vi "DefesaAntigaAdaptada.vi"(0 "Our Robot":T1={"id"=0, "function"=enum."Attacker", "x"=0.0, "y"=0.0, "orientation"=0.0, "v_tangent"=0.0, "v_normal"=0.0, "v_ang"=0.0, "kick_x"=0.0, "kick_z"=0.0, "dribble"=FALSE, "Timestamp"=timestamp(0 s since 1904-01-01), "estimatives"={"est_v_tangent"=0.0, "est_v_normal"=0.0, "est_vx"=0.0, "est_vy"=0.0, "Pos Robot Est"=[]}, "dest_x_kick"=0.0, "dest_y_kick"=0.0, "Gap Coord"=[], "States"=enum."GoToTangent", "Path "=[], "Path  Smooth"=[], "Dest"=[]}, 1 "total de \ndefensores":i32, 2 "Id duelist":u32, 3 "Stop?":bool=TRUE, 4 "AI Parameters":T12={"GotoKick"={"Dist do cone a frente"=150.0, "attacker farback"=1500.0, "Perto"=300.0, "min dist to kick"=150.0, "kick eps"=0.0, "Time to transition"=0.05}, "Attacker"={"CC chute"=0.09, "CC passe"=0.045, "Kick Force"=100.0, "ball-robot Kick"=200.0, "ball-robot Pass"=0.3, "drible\nAttk"=FALSE}, "Defender"={"D max"=1700.0, "Vel p/ robô av"=1000.0, "Kick Force"=100.0, "D atk-def"=0.0, "D farback"=0.0, "drible\ndef"=FALSE, "drible\ngoalie"=FALSE}, "Timeout"={"Field/v in x"=6.0, "Dist Robots"=300, "Dist up in y"=300}, "Pose Striker"={"dist"=200.0, "Numeric"=-4.0, "dist 2"=200.0, "drible\nstriker"=FALSE}, "Dist Stop"=300.0, "D ball out"=200, "D central gap "=150.0, "T pass"=0.0, "Force ++"=0.0, "range kick"=0.0, "Chute alto"=TRUE, "Marcador novo"=TRUE, "drible"=FALSE, "D drible"=300.0, "Versão Striker"=enum."Auto", "Defesa"=enum."ManMark", "Marcador"=enum."Marcar Segndo mais perigoso", "Receptor passe"=enum."Auto", "Área"=enum."Quadrada"} {"D drible" format="%#_13g"; "D central gap" format="%#_13g"; "Dist Stop" format="%#_13g"; "Pose Striker"."Numeric" format="%#_13g"; "Defender"."Kick Force" format="%#_13g"; "Defender"."Vel p/ robô av" format="%#_13g"; "Attacker"."ball-robot Kick" format="%#_13g"; "Attacker"."Kick Force" format="%#_13g"; "Attacker"."CC passe" format="%#_13g"; "Attacker"."CC chute" format="%#_13g"; "GotoKick"."kick eps" format="%#_13g"; "GotoKick"."min dist to kick" format="%#_13g"; "GotoKick"."Perto" format="%#_13g"; "GotoKick"."attacker farback" format="%#_13g"; "GotoKick"."Dist do cone a frente" format="%#_13g"}, 5 "balls":T7[](array[typedef]), 9 "geometry":T8, 10 "Atacando contra?":bool=TRUE, 11 "Field defense":dbl[](array[numeric]), 12 "Defensores":u32[](array[numeric]), 14 "IA State Input 2":T6={"our_robots"=[], "enemy_robots"=[], "balls"=[], "geometry"={"line_width"=0, "field_length"=0, "field_width"=0, "boundary_width"=0, "referee_width"=0, "goal_width"=0, "goal_depth"=0, "goal_wall_width"=0, "center_circle_radius"=0, "defense_radius"=0, "defense_stretch"=0, "free_kick_from_defense_dist"=0, "penalty_spot_from_field_line_dist"=0, "penalty_line_from_spot_dist"=0}, "IA Judge"={"stage"="", "command"="", "our_goalie_id"=0.0, "enemy_goalie_id"=0.0, "command enum"=enum."Halt", "Time"=enum."Azul"}, "Received Timestamp"=timestamp(0 s since 1904-01-01), "Events"={"Touch"=FALSE, "Ball out"=FALSE, "id touch"=0.0, "Ball out of \nVision"=FALSE, "Ball inside \nGoalie area"=FALSE, "Robot not responding"=FALSE, "Robots responding status"=[1.0, 1.0, 1.0, 1.0, 1.0, 1.0], "Enemy Ball \nPossession"=FALSE, "Pass State"=FALSE, "id end of pass"=0.0, "Kick"=FALSE, "Id ini Possession"=0.0, "Ball Possesion"=FALSE, "Id Possesion"=0.0, "Direct Kick"=FALSE, "2nd Strk Ativo"=FALSE}}) -> (6 "Robot out":T1={"id"=0, "function"=enum."Attacker", "x"=0.0, "y"=0.0, "orientation"=0.0, "v_tangent"=0.0, "v_normal"=0.0, "v_ang"=0.0, "kick_x"=0.0, "kick_z"=0.0, "dribble"=FALSE, "Timestamp"=timestamp(0 s since 1904-01-01), "estimatives"={"est_v_tangent"=0.0, "est_v_normal"=0.0, "est_vx"=0.0, "est_vy"=0.0, "Pos Robot Est"=[]}, "dest_x_kick"=0.0, "dest_y_kick"=0.0, "Gap Coord"=[], "States"=enum."GoToTangent", "Path "=[], "Path  Smooth"=[], "Dest"=[]})   [LabVIEW 2017]
uses:
  AI Parameters.ctl
  Core/AI Robot.ctl
  Functions Enum.ctl
  AttackerStates.ctl
  Path Planning/RRT/PathDests.ctl
  Path Planning/RRT/PathDest.ctl
  Core/Field Size.ctl
  Core/AI Ball.ctl
  Core/AI Input.ctl
  Core/AI Judge.ctl
  Command Enum.ctl
  Util/Events/Events.ctl
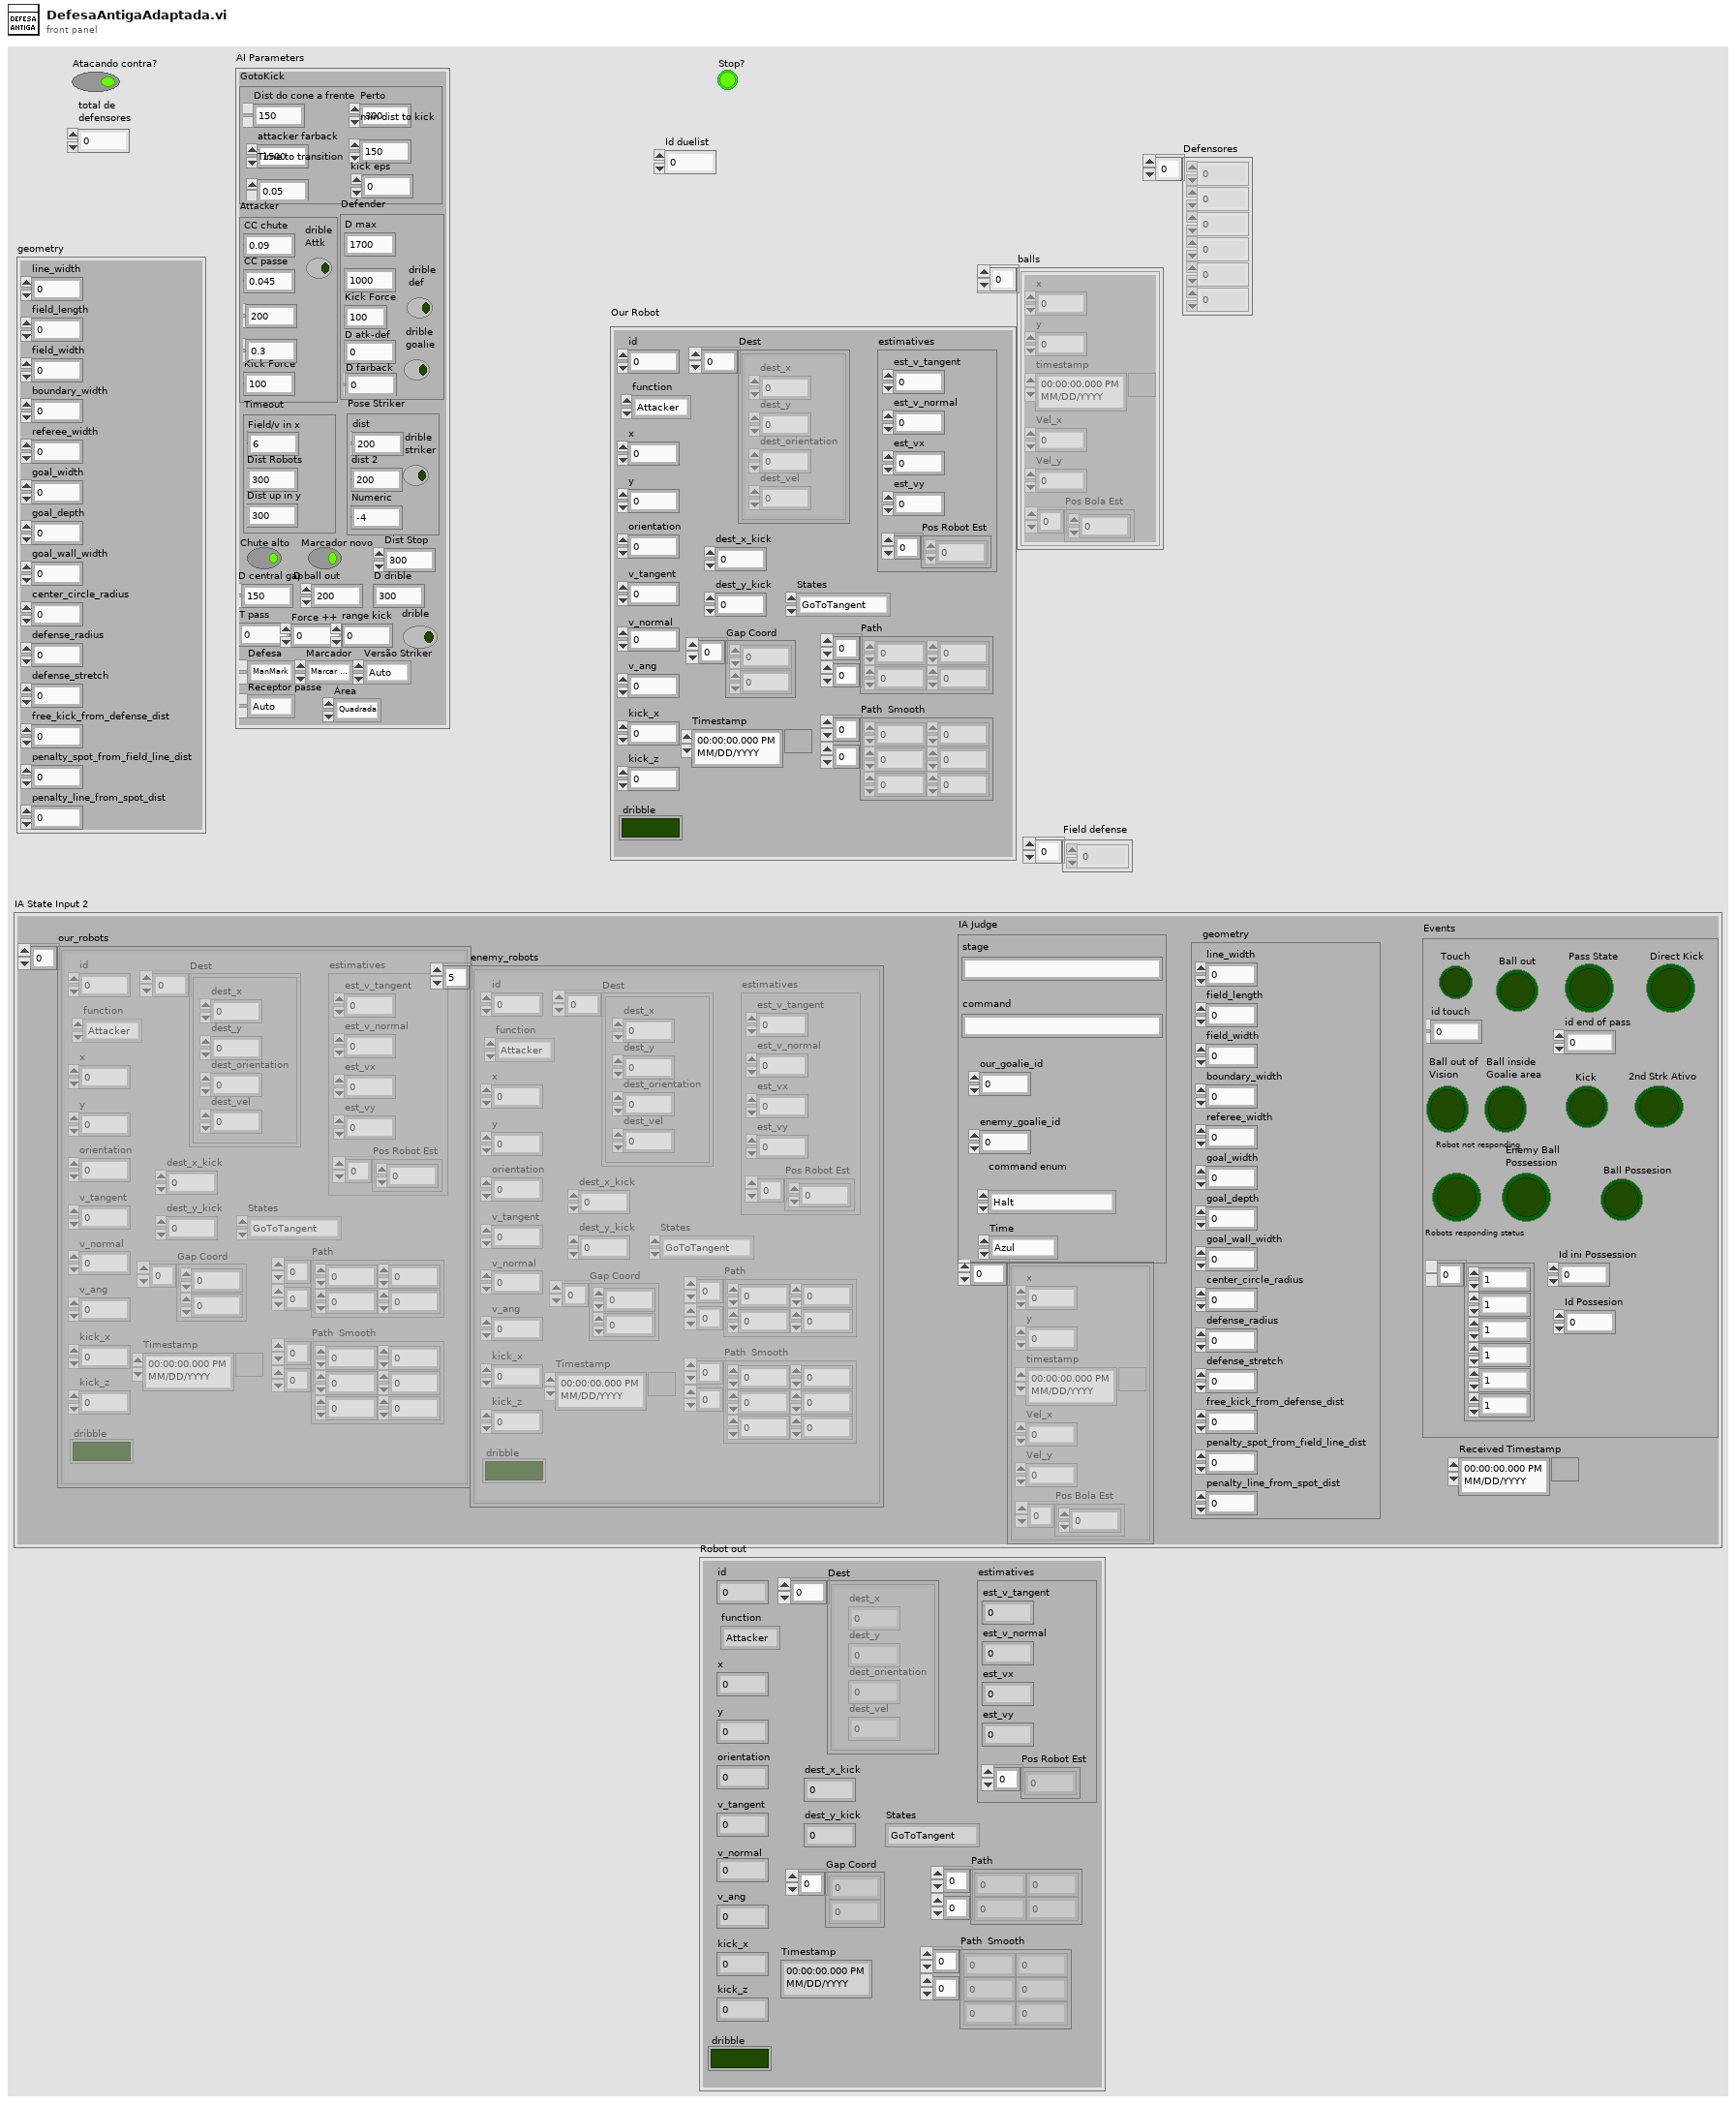
[diagram p1: front panel]
types:
  T1 = typedef "AI Robot.ctl" = cluster{"id":u32, "function":T2, "x":dbl, "y":dbl, "orientation":dbl, "v_tangent":dbl, "v_normal":dbl, "v_ang":dbl, "kick_x":dbl, "kick_z":dbl, "dribble":bool, "Timestamp":timestamp, "estimatives":cluster{"est_v_tangent":dbl, "est_v_normal":dbl, "est_vx":dbl, "est_vy":dbl, "Pos Robot Est":dbl[]}, "dest_x_kick":dbl, "dest_y_kick":dbl, "Gap Coord":dbl[], "States":T3, "Path ":dbl[][], "Path  Smooth":dbl[][], "Dest":T4}
  T2 = typedef "Functions Enum.ctl" = enum16{"2nd Striker", "Attacker", "Goalie", "Defender", "Striker", "Goto 0", "Dummy", "Kicker", "ZigZag 0", "ZigZag 1", "ZigZag 2", "ZigZag 3", "ZigZag 4", "ZigZag 5", "ZigZag 6", "ZigZag 7", "ZigZag 8", ""}
  T3 = typedef "AttackerStates.ctl" = enum16{"Pass", "GoToTangent", "BallGetting", "GoToKick", ""}
  T4 = typedef "PathDests.ctl" = T5[]
  T5 = typedef "PathDest.ctl" = cluster{"dest_x":dbl, "dest_y":dbl, "dest_orientation":dbl, "dest_vel":dbl}
  T6 = typedef "AI Input.ctl" = cluster{"our_robots":T1[], "enemy_robots":T1[], "balls":T7[], "geometry":T8, "IA Judge":T9, "Received Timestamp":timestamp, "Events":T11}
  T7 = typedef "AI Ball.ctl" = cluster{"x":dbl, "y":dbl, "timestamp":timestamp, "Vel_x":dbl, "Vel_y":dbl, "Pos Bola Est":dbl[]}
  T8 = typedef "Field Size.ctl" = cluster{"line_width":u32, "field_length":u32, "field_width":u32, "boundary_width":u32, "referee_width":u32, "goal_width":u32, "goal_depth":u32, "goal_wall_width":u32, "center_circle_radius":u32, "defense_radius":u32, "defense_stretch":u32, "free_kick_from_defense_dist":u32, "penalty_spot_from_field_line_dist":u32, "penalty_line_from_spot_dist":u32}
  T9 = typedef "AI Judge.ctl" = cluster{"stage":string, "command":string, "our_goalie_id":dbl, "enemy_goalie_id":dbl, "command enum":T10, "Time":enum16{"Azul", "Amarelo"}}
  T10 = typedef "Command Enum.ctl" = enum16{"Halt", "Stop", "Force Start", "PKA Normal Start", "Prepare Kickoff Ally", "PKE Normal Start", "Prepare Kickoff Enemy", "Prepare Penalty Ally", "PPA Normal Start", "Prepare Penalty Enemy", "PPE Normal Start", "Direct Free Enemy", "Direct Free Ally", "Indirect Free Enemy", "Indirect Free Ally", "Timeout Enemy", "Timeout Ally", "Goal Enemy", "Goal Ally", "Ball Placement Enemy", "Ball Placement Ally", "Normal Half Time", "Extra Time Break", "Extra Half Time", "None", "Post Game"}
  T11 = typedef "Events.ctl" = cluster{"Touch":bool, "Ball out":bool, "id touch":dbl, "Ball out of \nVision":bool, "Ball inside \nGoalie area":bool, "Robot not responding":bool, "Robots responding status":dbl[], "Enemy Ball \nPossession":bool, "Pass State":bool, "id end of pass":dbl, "Kick":bool, "Id ini Possession":dbl, "Ball Possesion":bool, "Id Possesion":dbl, "Direct Kick":bool, "2nd Strk Ativo":bool}
  T12 = typedef "AI Parameters.ctl" = cluster{"GotoKick":cluster{"Dist do cone a frente":dbl, "attacker farback":dbl, "Perto":dbl, "min dist to kick":dbl, "kick eps":dbl, "Time to transition":dbl}, "Attacker":cluster{"CC chute":dbl, "CC passe":dbl, "Kick Force":dbl, "ball-robot Kick":dbl, "ball-robot Pass":dbl, "drible\nAttk":bool}, "Defender":cluster{"D max":dbl, "Vel p/ robô av":dbl, "Kick Force":dbl, "D atk-def":dbl, "D farback":dbl, "drible\ndef":bool, "drible\ngoalie":bool}, "Timeout":cluster{"Field/v in x":dbl, "Dist Robots":u32, "Dist up in y":u32}, "Pose Striker":cluster{"dist":dbl, "Numeric":dbl, "dist 2":dbl, "drible\nstriker":bool}, "Dist Stop":dbl, "D ball out":i32, "D central gap ":dbl, "T pass":dbl, "Force ++":dbl, "range kick":dbl, "Chute alto":bool, "Marcador novo":bool, "drible":bool, "D drible":dbl, "Versão Striker":enum16{"Auto", "3", "2", "1"}, "Defesa":enum16{"ManMark", "Barreira"}, "Marcador":enum16{"Marcar Segndo mais perigoso", "Marcar o mais perigoso"}, "Receptor passe":enum16{"Auto", "2nd Striker", "Striker"}, "Área":enum16{"Quadrada", "Circular"}}
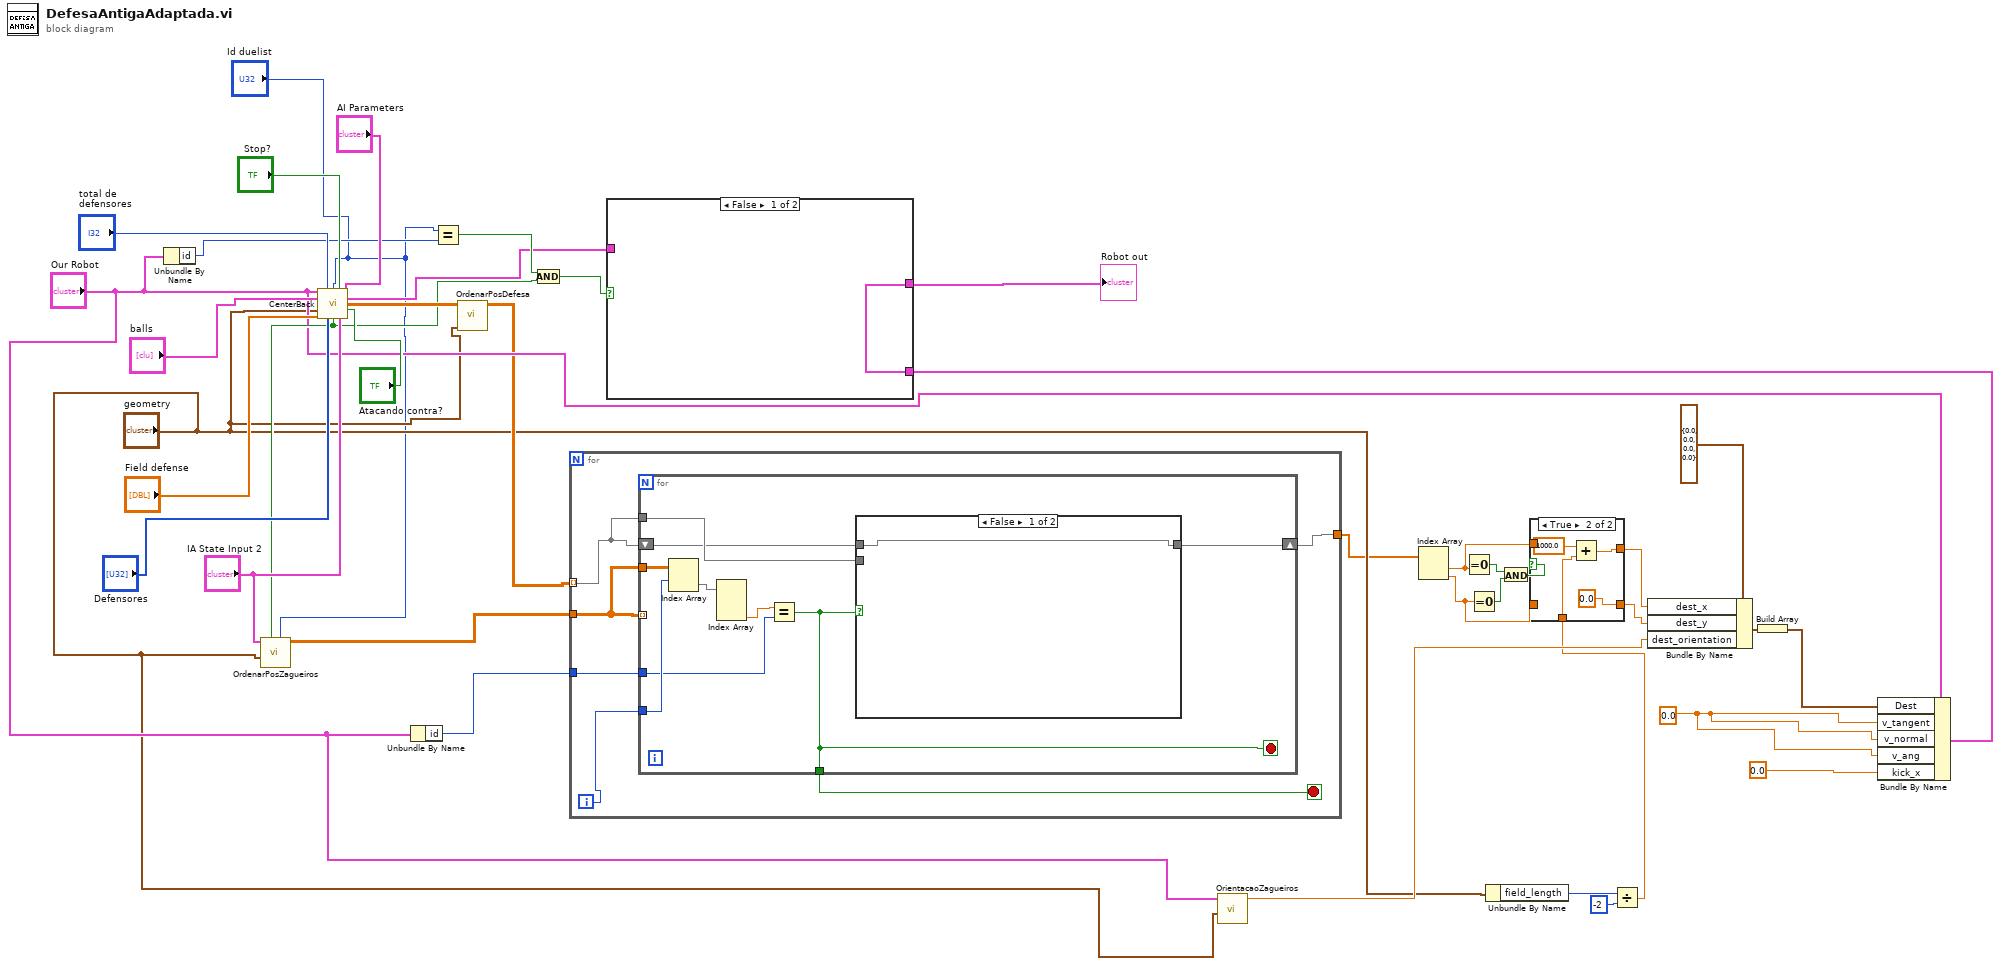
[diagram p0: block diagram]
diagram:
  w17 = 0.0
  n1 = Unbundle By Name("Our Robot") -> ("id"=w31:u32)
  n2 = call "CenterBack.vi"("Our Robot in"="Our Robot", "total"="total de \ndefensores", "Id duelist"="Id duelist", "Stop?"="Stop?", "AI Parameters"="AI Parameters", "balls"="balls", "Field Size in"="geometry", "Atacando contra?"="Atacando contra?", "Field defense"="Field defense", "Defensores"="Defensores", "IA State Input 2"="IA State Input 2") -> ("Robot out"=w27:T1, "Pos Centers Back"=w39:dbl[][], "Zageuiro duelist?"=w25:bool)  [unwired: 2 in]
  n3 = call "OrdenarPosZagueiros.vi"("ID duelist"="Id duelist", "Zagueiro duelist?"=w25, "geometry"="geometry", "IA State Input 2"="IA State Input 2") -> ("Posições ordenadas zagueiros"=w15:dbl[][])  [unwired: 7 in]
  n4 = Unbundle By Name("Our Robot") -> ("id"=w14:u32)
  n5 = Equal?(x="Id duelist", y=w31) -> (x = y?=w30:bool)
  n6 = call "OrdenarPosDefesa.vi"("geometry"="geometry", "Posições da defesa"=w39) -> ("Posições ordenadas"=w16:dbl[][])  [unwired: 9 in]
  n7 = And(x=w30, y=w25) -> (x .and. y?=w29:bool)
  n8 = for {
    tunnel: w16 -> [w42] mode=indexing
    tunnel: w15 -> [w44]
    tunnel: w14 -> [w45]
    tunnel: [w41] -> w2
    i -> [w43]
    stop <- w40 stop-if-true
    n9 = for {
      tunnel: w44 -> [_] mode=indexing
      tunnel: w45 -> [w50]
      tunnel: w44 -> [w54]
      tunnel: w43 -> [w53]
      shift-right: [w48] -> w41
      shift-left: w42 -> [w47]
      tunnel: w42 -> [w49]
      tunnel: [w46] -> w40
      stop <- w46 stop-if-true
      n10 = Index Array(array=w54, index (row)=w53) -> (element=w52:dbl[])  [unwired: 1 in]
      n11 = Index Array(array=w52) -> (element #3=w51:dbl)  [unwired: 3 in, 2 out]
      n12 = Equal?(x=w51, y=w50) -> (x = y?=w46:bool)
      n13 = case shown="False" w46 {
        tunnel: w49 -> [_ w56]
        tunnel: [w55 w56] -> w48
        tunnel: w47 -> [w55 _]
        frame False {
        }
        frame True {
        }
      }
    }
  }
  n14 = call "OrientacaoZagueiros.vi"("geometry"="geometry", "Our Robot"="Our Robot") -> ("Orientação Center Back"=w18:dbl)  [unwired: 9 in]
  n15 = Index Array(array=w2) -> (element #1=w9:dbl, element #2=w7:dbl)  [unwired: 2 in]
  n16 = Equal To 0?(x=w9) -> (x = 0?=w13:bool)
  n17 = Equal To 0?(x=w7) -> (x = 0?=w12:bool)
  n18 = Unbundle By Name("geometry") -> ("field_length"=w5:u32)
  n19 = And(x=w13, y=w12) -> (x .and. y?=w11:bool)
  n20 = Divide(x=w5, y=-2) -> (x/y=w3:dbl)
  n21 = case shown="True" w11 {
    tunnel: [w58 w59] -> w10
    tunnel: w9 -> [w58 _]
    tunnel: [w57 0.0] -> w8
    tunnel: w7 -> [w57 _]
    tunnel: w3 -> [_ w61]
    frame False {
    }
    frame True {
      n22 = Add(x=1000.0, y=w61) -> (x+y=w59:dbl)
    }
  }
  n23 = Bundle By Name(cluster=T5 {"dest_x"=0.0, "dest_y"=0.0, "dest_orientation"=0.0, "dest_vel"=0.0} ("element"), "dest_x"=w10, "dest_y"=w8, "dest_orientation"=w18) -> (w24:T5)
  n24 = Build Array(w24) -> (w23:T5[])
  n25 = Bundle By Name(cluster="Our Robot", "Dest"=w23, "v_tangent"=w17, "v_normal"=w17, "v_ang"=w17, "kick_x"=0.0) -> (w20:T1)
  n26 = case shown="False" w29 {
    tunnel: [w63 w64] -> w28
    tunnel: w27 -> [_ w64]
    tunnel: w20 -> [w63 _]
    frame False {
    }
    frame True {
    }
  }
  "Robot out" <- w28
